vi "1003_FireAt1015SpecificYear.vi"(8 "error in (no error)":errorcluster) -> (0 "error out":errorcluster)   [LabVIEW 2013]
uses:
  <vilib>/addons/_JKI Toolkits/Caraya/classes/Assert/Assert True.vi
  source/Cron/Create Cron Job.vi
  source/Cron/Compute Next Cron.vi
  source/Cron.Unix/Cron.Unix.lvclass
  <vilib>/addons/_JKI Toolkits/Caraya/classes/Test/Test.lvclass
  <vilib>/addons/_JKI Toolkits/Caraya/classes/Assert/Assert.lvclass
  source/openCron.lvlib
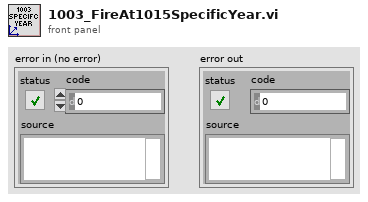
[diagram p1: front panel]
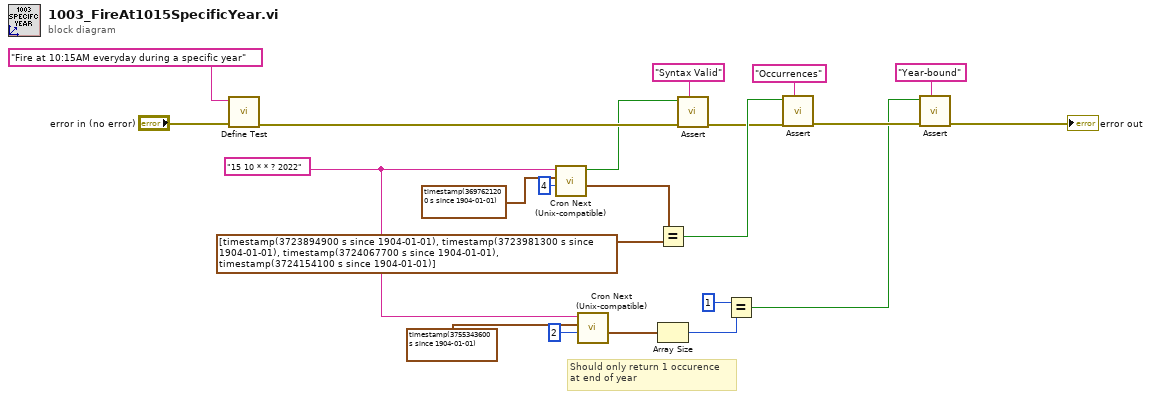
[diagram p0: block diagram]
diagram:
  w4 = "15 10 * * ? 2022" ("Expression")
  # "Should only return 1 occurence\nat end of year"
  n1 = call <vilib>:"Define Test.vi"("error in (no error)"="error in (no error)", "Label (VI Title)"="Fire at 10:15AM everyday during a specific year") -> ("error out"=w19:errorcluster)  [unwired: 9 in]
  n2 = call "Cron Next (Unix-compatible).vi"("Nb Occurences (min: 1)"=u16 4, "Reference timestamp (Now)"=timestamp(3697621200 s since 1904-01-01) ("y"), "Cron Expression"=w4) -> ("Occurences"=w6:timestamp[], "syntax valid?"=w5:bool)  [unwired: 6 in, 1 out]
  n3 = call "Cron Next (Unix-compatible).vi"("Nb Occurences (min: 1)"=u16 2, "Reference timestamp (Now)"=timestamp(3755343600 s since 1904-01-01) ("y"), "Cron Expression"=w4) -> ("Occurences"=w1:timestamp[])  [unwired: 6 in, 2 out]
  n4 = Equal?(x=w6, y=timestamp[] [timestamp(3723894900 s since 1904-01-01), timestamp(3723981300 s since 1904-01-01), timestamp(3724067700 s since 1904-01-01), timestamp(3724154100 s since 1904-01-01)]) -> (x = y?=w18:bool)
  n5 = Array Size(array=w1) -> (size(s)=w11:i32)
  n6 = call-poly <vilib>:"Assert.vi"("Label"="Syntax Valid" ("Label (VI Title)"), "error in (no error)"=w19, "True?"=w5) -> ("error out"=w17:errorcluster)  [unwired: 8 in]
  n7 = Equal?(x=1, y=w11) -> (x = y?=w9:bool)
  n8 = call-poly <vilib>:"Assert.vi"("Label"="Occurrences" ("Label (VI Title)"), "error in (no error)"=w17, "True?"=w18) -> ("error out"=w13:errorcluster)  [unwired: 8 in]
  n9 = call-poly <vilib>:"Assert.vi"("Label"="Year-bound" ("Label (VI Title)"), "error in (no error)"=w13, "True?"=w9) -> ("error out"=→"error out":errorcluster)  [unwired: 8 in]
